vi "两个数据比较.vi"(8 "误差":sgl, 10 "标准值":sgl, 11 "实际值":sgl) -> (2 "相等?":bool)   [LabVIEW 2010]
panel:
  # "0~1"
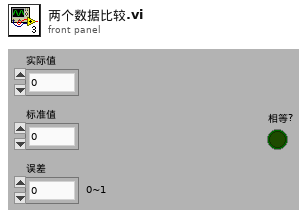
[diagram p1: front panel]
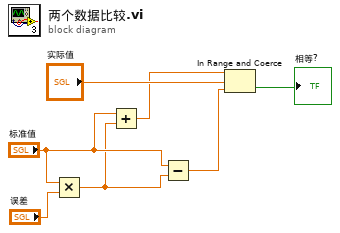
[diagram p0: block diagram]
diagram:
  n1 = Multiply(x="标准值", y="误差") -> (x*y=w4:sgl)
  n2 = Add(x="标准值", y=w4) -> (x+y=w3:sgl)
  n3 = Subtract(x="标准值", y=w4) -> (x-y=w2:sgl)
  n4 = In Range and Coerce(upper limit=w3, x="实际值", lower limit=w2) -> (In Range?=→"相等?":bool)  [unwired: 1 out]
